vi "Convert_ERDs.vi"(0 "New Header?":bool, 2 "ERD Name":string[](array[string]), 5 "All_Bundled_Data_Brass":T1, 7 "Array":T8[](array[typedef]) {"ERD Number" format="%.0x"}, 11 "Error In":errorcluster) -> (6 "All_ERD_Data_Bundled_Brass":T1, 15 "Error Out":errorcluster)   [LabVIEW 2021]
doc: "This VI parses the data from ERDs in correct format, units, etc. It handles all hex to dec conversions, hex to enum, and hex to boolean conversions.\n\nIf Raw Data from ERD is blank string, then it will output values from shift register."
uses:
  Common/LabVIEW GEA2 Toolkit/GEA3/type defs/ERD Read Data Out.ctl
  Controls/All_Bundled_Data_RT.ctl
  Dryer Tool (Commercial 2)/JL Dryer Tool Support/type defs/Version.ctl
  Dryer Tool (Commercial 2)/JL Dryer Tool Support/type defs/ERD_Always_Show_JL.ctl
  Dryer Tool (Commercial 2)/JL Dryer Tool Support/type defs/CSV_File_String_Arrays.ctl
  Dryer Tool (Commercial 2)/JL Dryer Tool Support/type defs/Fault Table Array.ctl
  Dryer Tool (Commercial 2)/JL Dryer Tool Support/type defs/Fault_Table_Info.ctl
  Dryer Tool (Commercial 2)/JL Dryer Tool Support/type defs/BootloaderVersion.ctl
panel:
  out "Numeric":i32
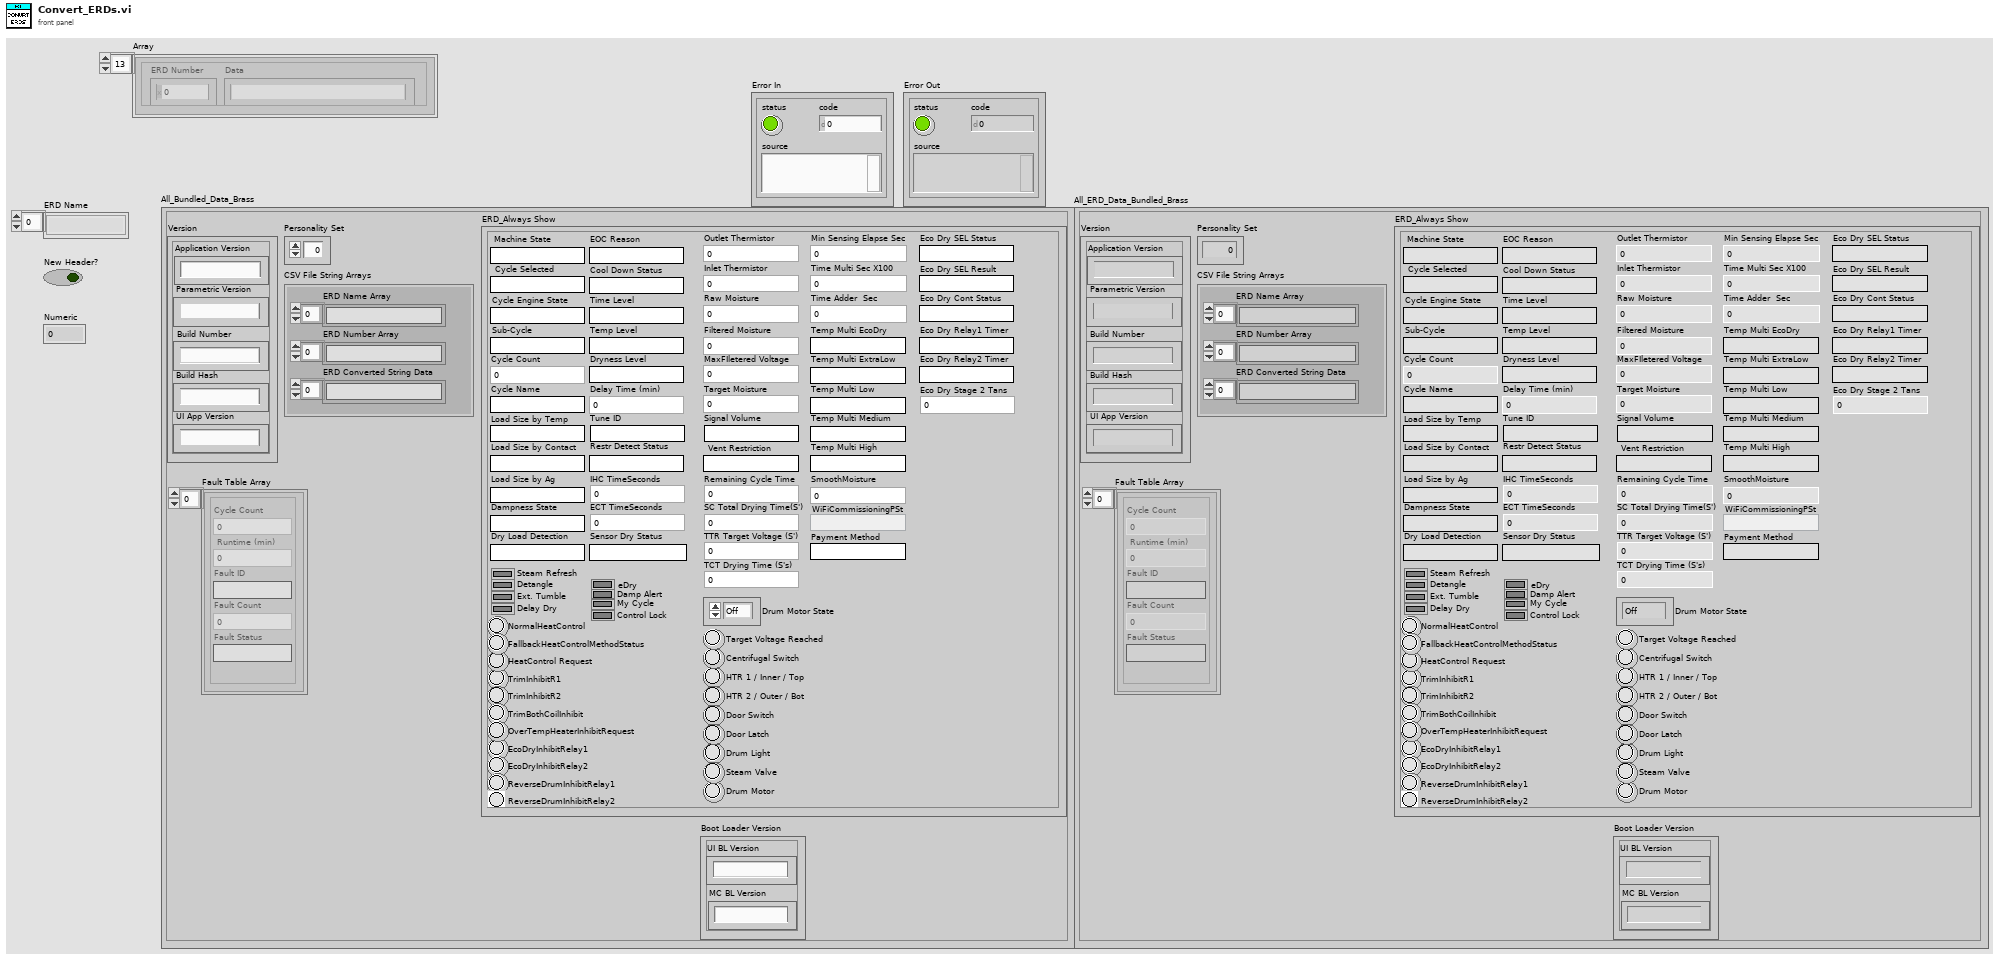
[diagram p1: front panel]
types:
  T1 = typedef "All_Bundled_Data_RT.ctl" = cluster{"Version":T2, "ERD_Always Show":T3, "Personality Set":u8, "CSV File String Arrays":T4, "Fault Table Array ":T5, "Boot Loader Version":T7}
  T2 = typedef "Version.ctl" = cluster{"Build Number":string, "Build Hash ":string, "Application Version":string, "Parametric Version":string, "UI App Version":string}
  T3 = typedef "ERD_Always_Show_JL.ctl" = cluster{"Inlet Thermistor":u16, "Machine State":string, "Filtered Moisture":u16, "Cycle Selected":string, "HTR 1 / Inner / Top":bool, "HTR 2 / Outer / Bot":bool, "Door Switch":bool, "Drum Light":bool, "Cycle Engine State":string, "Centrifugal Switch":bool, "Drum Motor":bool, "Cycle Count":u32, "Ext. Tumble":bool, "eDry":bool, "Temp Level":string, "Dryness Level":string, "Time Level":string, "Delay Time (min)":u16, "Steam Refresh":bool, "Damp Alert":bool, "Sub-Cycle":string, "Outlet Thermistor":u16, "Target Moisture":u16, "Remaining Cycle Time":u32, "Raw Moisture":u16, "Cycle Name":string, "My Cycle":bool, "Delay Dry":bool, "Detangle":bool, "Control Lock":bool, "Steam Valve":bool, "Door Latch":bool, "Signal Volume":string, "Tune ID":string, "Restr Detect Status":string, "Vent Restriction":string, "Load Size by Contact":string, "Load Size by Temp":string, "EOC Reason":string, "Sensor Dry Status":string, "Dampness State":string, "Target Voltage Reached":bool, "TrimInhibitR1":bool, "TrimInhibitR2":bool, "TrimBothCoilInhibit":bool, "NormalHeatControl":bool, "HeatControl Request":bool, "Cool Down Status":string, "EcoDryInhibitRelay1":bool, "EcoDryInhibitRelay2":bool, "ReverseDrumInhibitRelay1":bool, "ReverseDrumInhibitRelay2":bool, "OverTempHeaterInhibitRequest":bool, "FallbackHeatControlMethodStatus":bool, "IHC TimeSeconds":u32, "ECT TimeSeconds ":u32, "SC Total Drying Time(S')":u32, "TTR Target Voltage (S')":u32, "TCT Drying Time (S's)":u32, "Drum Motor State":enum16{"Off", "Cw", "Ccw", "Max"}, "Load Size by Ag":string, "MaxFIletered Voltage":u16, "Dry Load Detection":string, "Min Sensing Elapse Sec":u32, "Time Multi Sec X100":u32, "Time Adder  Sec":u32, "Temp Multi EcoDry":string, "Temp Multi ExtraLow":string, "Temp Multi Low ":string, "Temp Multi Medium":string, "Temp Multi High":string, "SmoothMoisture":u16, "Eco Dry SEL Status":string, "Eco Dry SEL Result":string, "Eco Dry Cont Status":string, "Eco Dry Relay1 Timer":string, "Eco Dry Relay2 Timer ":string, "Eco Dry Stage 2 Tans ":u32, "WiFiCommissioningPSt":string, "Payment Method":string}
  T4 = typedef "CSV_File_String_Arrays.ctl" = cluster{"ERD Number Array":string[], "ERD Name Array":string[], "ERD Converted String Data":string[]}
  T5 = typedef "Fault Table Array.ctl" = T6[]
  T6 = typedef "Fault_Table_Info.ctl" = cluster{"Cycle Count":u32, " Runtime (min) ":u32, "Fault Status":string, "Fault ID":string, "Fault Count":u16}
  T7 = typedef "BootloaderVersion.ctl" = cluster{"UI BL Version":string, "MC BL Version":string}
  T8 = typedef "ERD Read Data Out.ctl" = cluster{"ERD Number":u16, "Data":string}
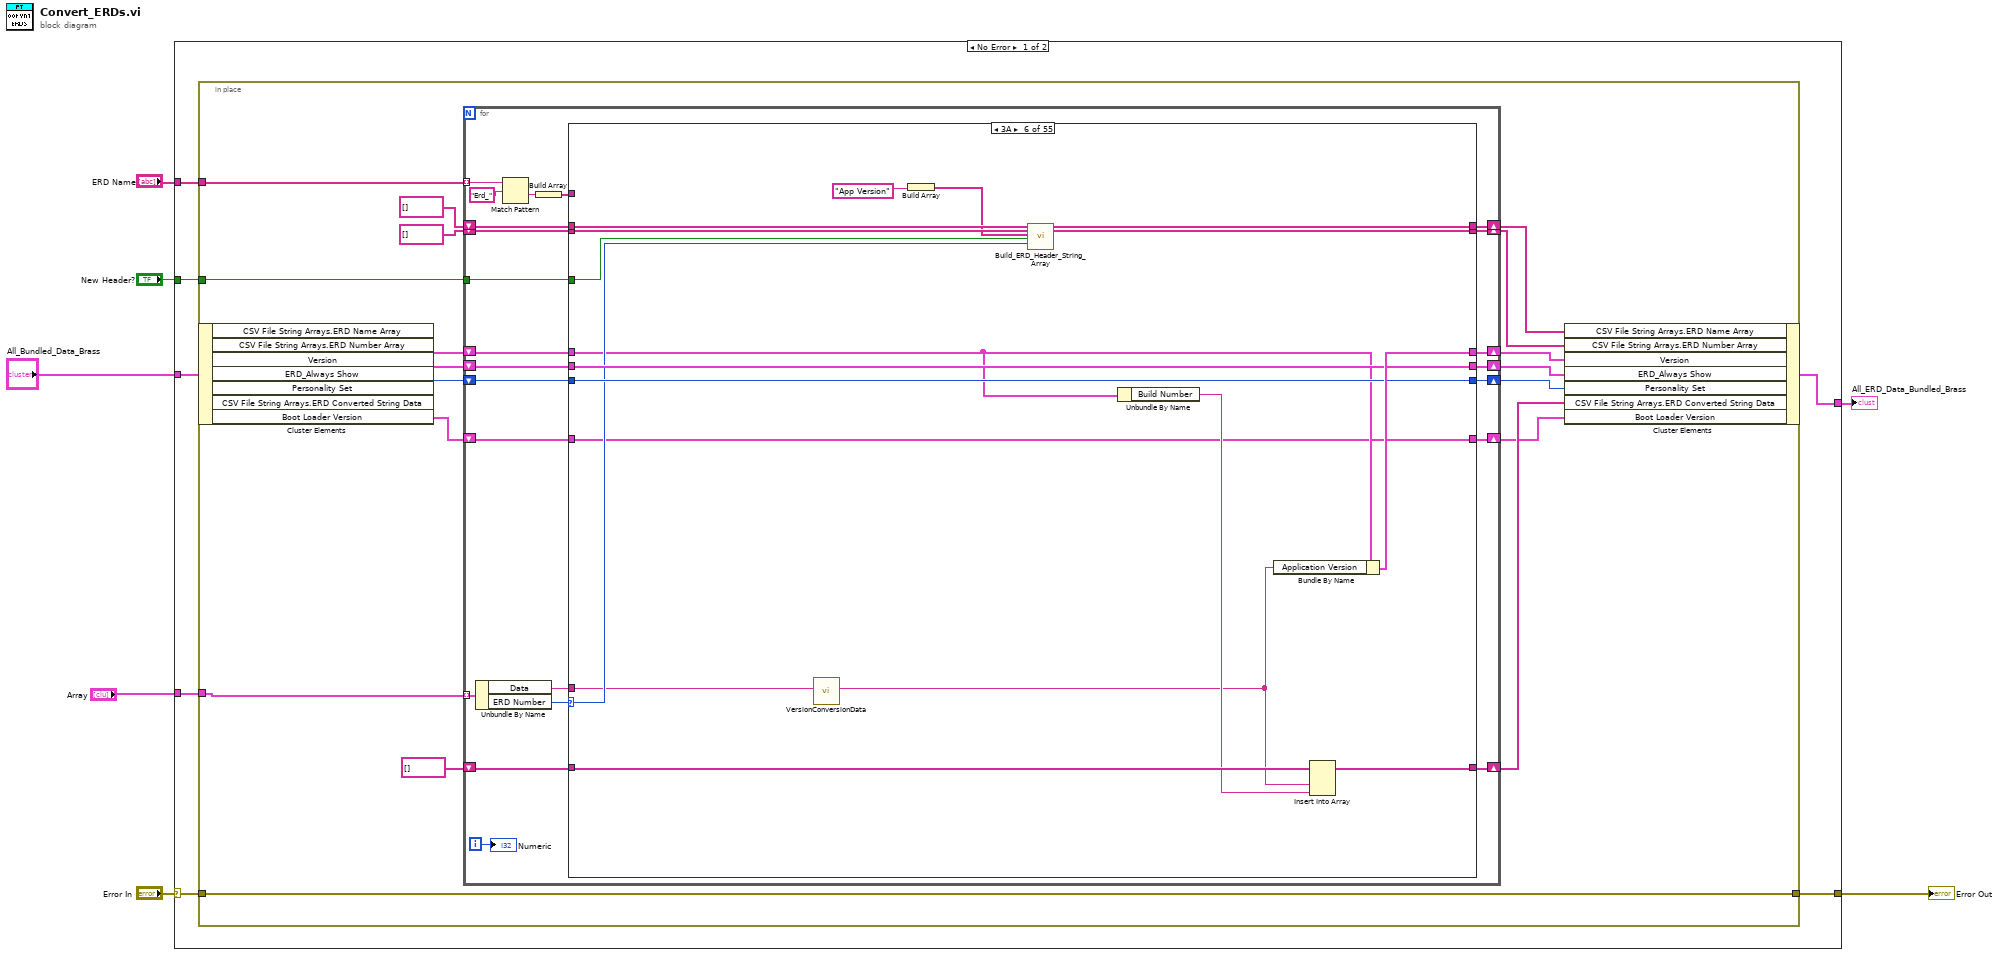
[diagram p0: block diagram]
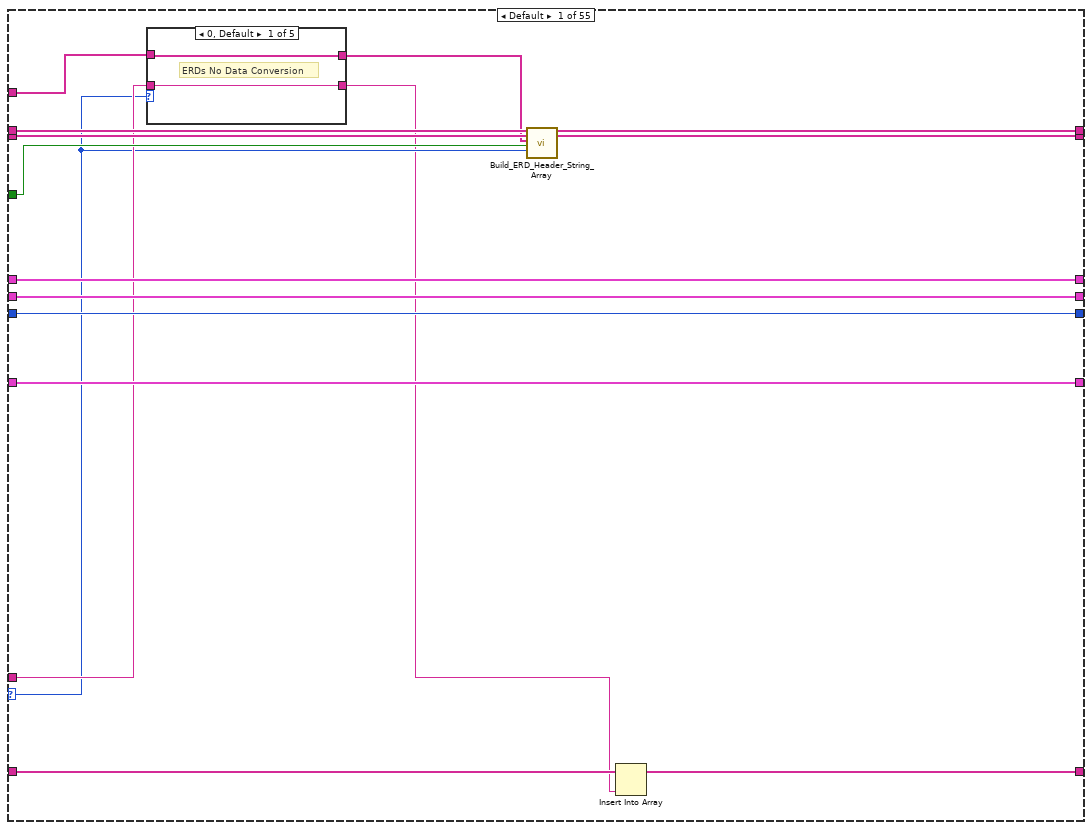
[diagram p2: hidden frame]
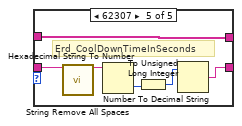
[diagram p6: hidden frame]
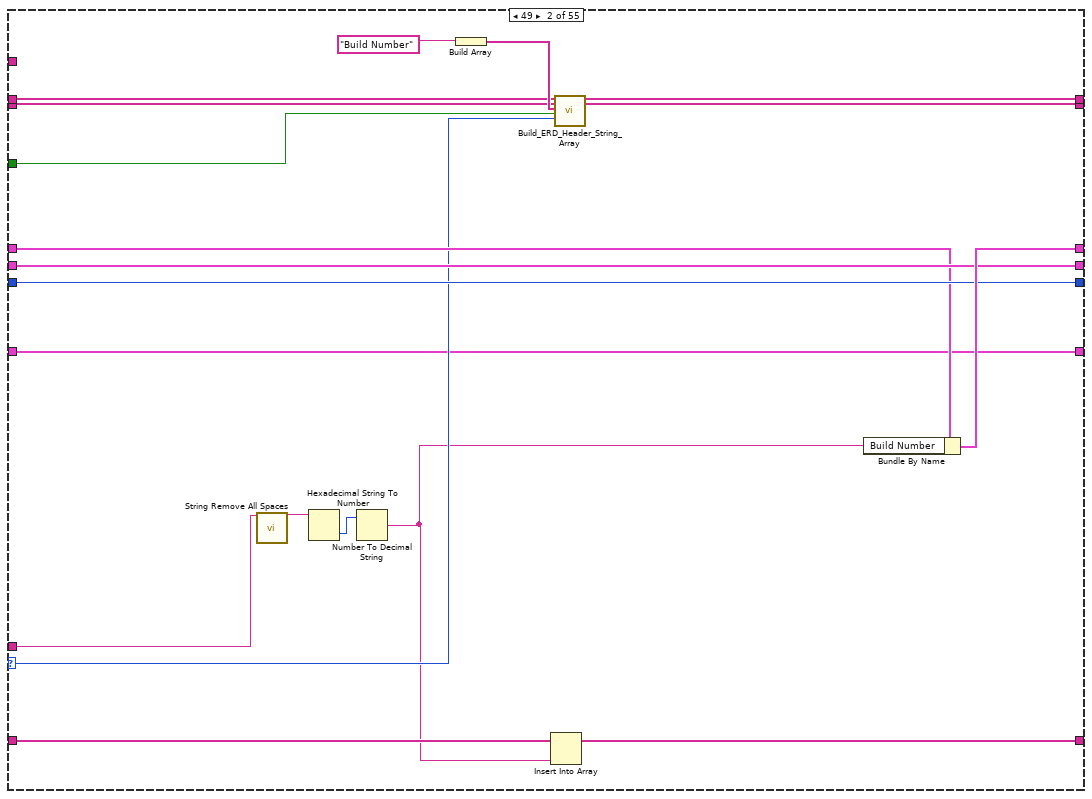
[diagram p7: hidden frame]
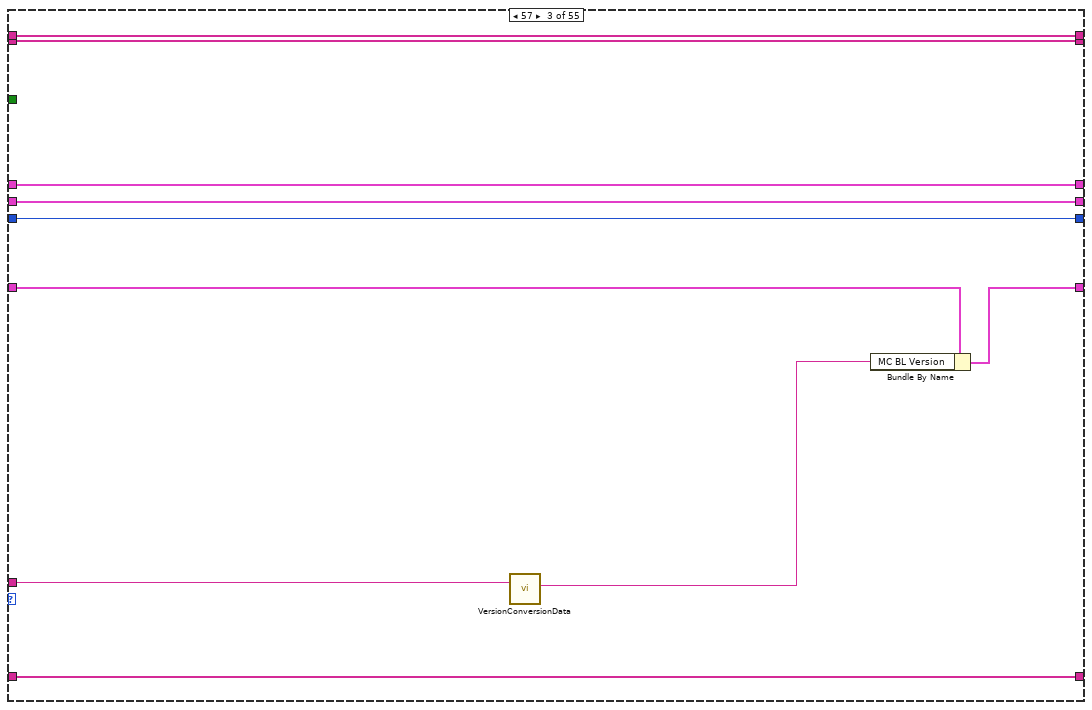
[diagram p8: hidden frame]
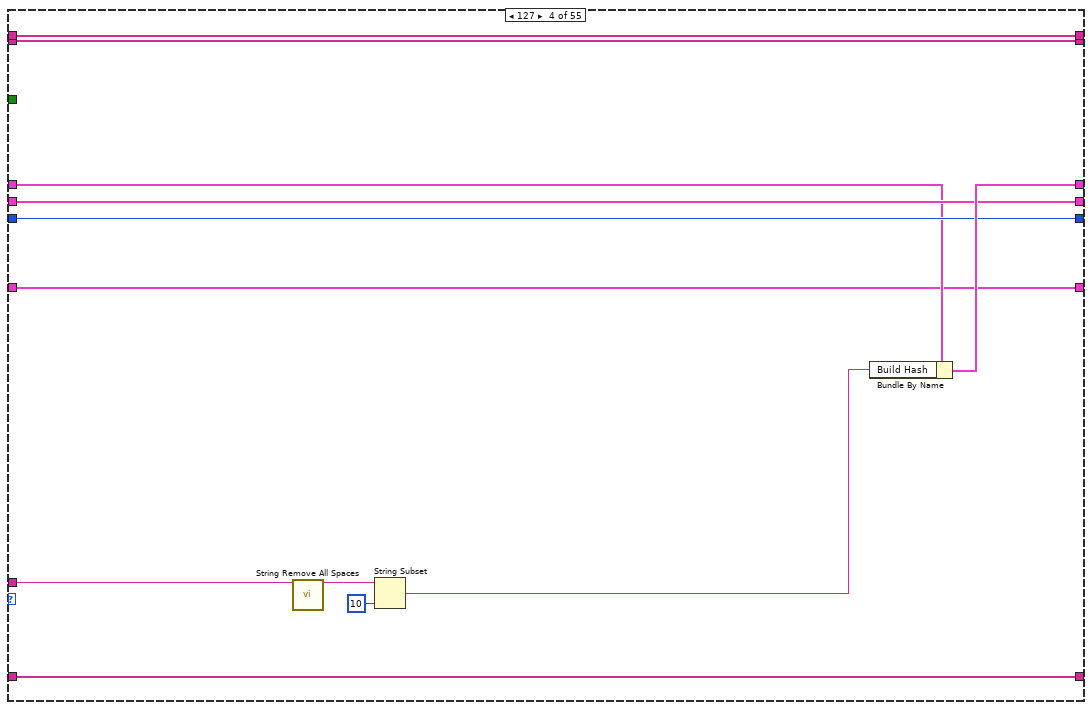
[diagram p9: hidden frame]
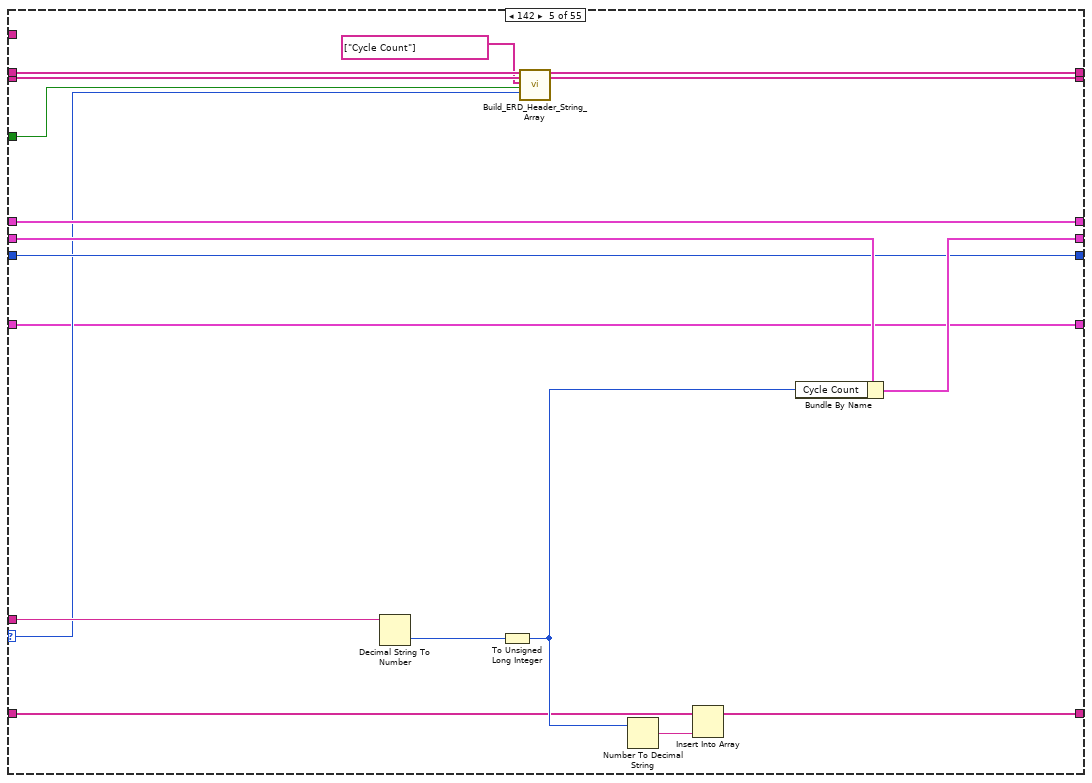
[diagram p10: hidden frame]
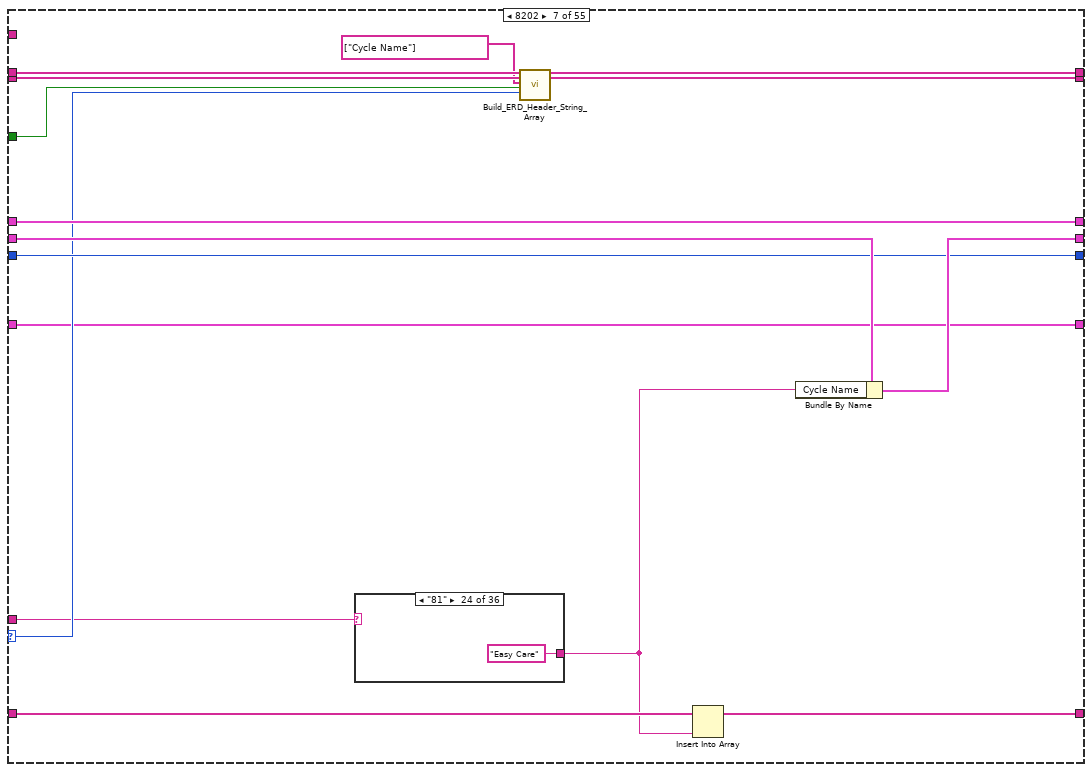
[diagram p11: hidden frame]
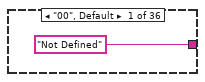
[diagram p12: hidden frame]
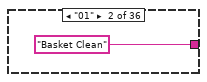
[diagram p13: hidden frame]
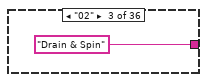
[diagram p14: hidden frame]
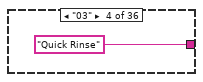
[diagram p15: hidden frame]
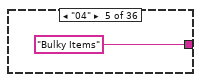
[diagram p16: hidden frame]
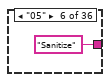
[diagram p17: hidden frame]
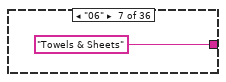
[diagram p18: hidden frame]
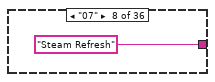
[diagram p19: hidden frame]
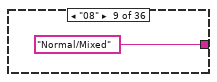
[diagram p20: hidden frame]
diagram:
  n1 = case shown="No Error" "Error In" {
    selector: "Error In" -> [w11 w1202]
    tunnel: "Array" -> [w14 _]
    tunnel: [w12 w1201] -> w5
    tunnel: "All_Bundled_Data_Brass" -> [w13 w1200]
    tunnel: [w10 w1200] -> w1
    tunnel: "New Header?" -> [w9 _]
    tunnel: "ERD Name" -> [w8 _]
    frame No Error {
      n2 = in-place {
        in-place-border: w14 -> [w16]
        in-place-border: [w15] -> w12
        in-place-border: w11 -> [w15]
        in-place-border: w9 -> [w25]
        in-place-border: w8 -> [w17]
        n3 = in-place-cluster #1(w13) -> ("Version"=w31:T2, "ERD_Always Show"=w32:T3, "Personality Set"=w28:u8, "Boot Loader Version"=w19:T7)  [unwired: 3 out]
        n4 = for {
          shift-right: [w54] -> w29
          shift-left: w32 -> [w53]
          shift-right: [w51] -> w30
          shift-left: w31 -> [w52]
          shift-right: [w48] -> w27
          shift-left: w28 -> [w49]
          shift-right: [w46] -> w20
          shift-left: string[] [] ("ERD String Data") -> [w47]
          tunnel: w25 -> [w45]
          shift-right: [w41] -> w21
          shift-left: string[] [] ("ERD String Data") -> [w44]
          shift-right: [w42] -> w22
          shift-left: string[] [] ("ERD String Data") -> [w43]
          shift-right: [w38] -> w18
          shift-left: w19 -> [w39]
          tunnel: w17 -> [w37] mode=indexing
          tunnel: w16 -> [w33] mode=indexing
          i -> [w40]
          n5 = Unbundle By Name(w33) -> ("Data"=w55:string, "ERD Number"=w50:u16)
          n6 = Match Pattern(string=w37, regular expression="Erd_") -> (after substring=w34:string)  [unwired: 1 in, 3 out]
          n7 = Build Array(w34) -> (w35:string[])
          n8 = case shown="3A" w50 {
            selector: w50 -> [w57 w95 _ _ w133 w154 w168 w223 w244 w276 w304 w322 w341 w360 w379 w398 w419 w442 w460 w471 w494 w526 w540 w556 w581 w600 w627 w650 w669 w690 w710 w729 w748 w766 w785 w808 w824 w849 w870 w889 w908 w927 w949 w975 w990 w1014 w1033 w1052 w1074 w1094 w1110 w1133 w1156 w1168 w1192]
            tunnel: w55 -> [w58 w89 w106 w120 w144 w146 w165 w217 w237 w275 w303 w320 w339 w358 w377 w396 w414 w437 w452 w473 w499 w522 w538 w569 w580 w611 w637 w664 w683 w700 w724 w743 w762 w779 w798 w819 w835 w859 w881 w900 w919 w938 w960 w970 w1000 w1013 w1032 w1051 w1085 w1088 w1121 w1131 w1153 w1166 w1184]
            tunnel: [w71 w103 w114 w125 w142 w161 w177 w231 w241 w288 w316 w336 w355 w374 w393 w412 w415 w433 w451 w479 w496 w520 w554 w568 w592 w612 w636 w662 w681 w699 w722 w741 w760 w780 w799 w817 w836 w860 w882 w901 w920 w939 w961 w984 w999 w1026 w1045 w1064 w1083 w1103 w1119 w1127 w1154 w1178 w1185] -> w54
            tunnel: w53 -> [w71 w103 w114 w125 w143 w161 w178 w231 w242 w289 w317 w333 w352 w371 w390 w409 w416 w434 w455 w478 w497 w521 w551 w570 w593 w613 w638 w663 w682 w701 w723 w742 w761 w781 w800 w818 w837 w861 w883 w902 w921 w940 w962 w985 w1001 w1027 w1046 w1065 w1084 w1104 w1120 w1128 w1155 w1178 w1186]
            tunnel: w52 -> [w70 w101 w107 w121 w141 w153 w176 w230 w243 w287 w315 w335 w354 w373 w392 w411 w428 w435 w466 w489 w512 w535 w553 w567 w591 w610 w635 w661 w680 w698 w721 w740 w759 w778 w797 w816 w834 w858 w880 w899 w918 w937 w959 w983 w998 w1025 w1044 w1063 w1082 w1102 w1118 w1141 w1164 w1180 w1196]
            tunnel: [w70 w104 w107 w126 w141 w162 w176 w230 w243 w287 w315 w335 w354 w373 w392 w411 w428 w435 w466 w489 w512 w535 w553 w567 w591 w610 w635 w661 w680 w698 w721 w740 w759 w778 w797 w816 w834 w858 w880 w899 w918 w937 w959 w983 w998 w1025 w1044 w1063 w1082 w1102 w1118 w1141 w1164 w1179 w1196] -> w51
            tunnel: w49 -> [w69 w102 w113 w124 w140 w160 w175 _ w251 w286 w314 w332 w351 w370 w389 w408 w427 w448 w465 w488 w511 w534 w550 w566 w590 w609 w634 w660 w679 w697 w720 w739 w758 w777 w796 w815 w833 w857 w879 w898 w917 w936 w958 w982 w997 w1024 w1043 w1062 w1081 w1101 w1117 w1140 w1163 w1177 w1195]
            tunnel: [w69 w102 w113 w124 w140 w160 w175 w219 w251 w286 w314 w332 w351 w370 w389 w408 w427 w448 w465 w488 w511 w534 w550 w566 w590 w609 w634 w660 w679 w697 w720 w739 w758 w777 w796 w815 w833 w857 w879 w898 w917 w936 w958 w982 w997 w1024 w1043 w1062 w1081 w1101 w1117 w1140 w1163 w1177 w1195] -> w48
            tunnel: w47 -> [w67 w99 w110 w116 w138 w149 w173 w227 w248 w281 w308 w326 w345 w364 w383 w402 w423 w444 w458 w482 w503 w530 w544 w560 w586 w606 w631 w654 w673 w694 w714 w733 w752 w771 w790 w812 w830 w855 w876 w895 w914 w933 w955 w979 w994 w1018 w1037 w1056 w1078 w1098 w1114 w1137 w1160 w1172 w1188]
            tunnel: [w63 w98 w110 w116 w136 w156 w171 w225 w246 w279 w306 w324 w343 w362 w381 w400 w421 w440 w461 w485 w502 w528 w542 w558 w584 w604 w629 w652 w671 w692 w712 w731 w750 w769 w788 w810 w828 w853 w874 w893 w912 w931 w953 w977 w992 w1016 w1035 w1054 w1076 w1096 w1112 w1135 w1158 w1170 w1190] -> w46
            tunnel: w45 -> [w65 w93 _ _ w134 w155 w169 w224 w245 w278 w305 w323 w342 w361 w380 w399 w420 w443 w459 w481 w500 w527 w541 w557 w583 w601 w628 w651 w670 w691 w711 w730 w749 w768 w787 w809 w825 w850 w871 w890 w909 w928 w950 w976 w991 w1015 w1034 w1053 w1075 w1095 w1111 w1134 w1157 w1169 w1193]
            tunnel: w44 -> [w66 w97 w111 w122 w139 w150 w174 w228 w249 w282 w309 w327 w346 w365 w384 w403 w424 w445 w457 w483 w504 w531 w545 w561 w587 w607 w632 w655 w674 w695 w715 w734 w753 w772 w791 w813 w831 w856 w877 w896 w915 w934 w956 w980 w995 w1019 w1038 w1057 w1079 w1099 w1115 w1138 w1161 w1173 w1189]
            tunnel: w43 -> [w61 w91 w112 w123 w129 w159 w167 w221 w234 w284 w312 w330 w349 w368 w387 w406 w418 w439 w453 w476 w498 w524 w548 w565 w589 w603 w626 w658 w677 w689 w718 w737 w756 w775 w794 w807 w827 w852 w873 w892 w911 w930 w952 w974 w989 w1022 w1041 w1060 w1072 w1092 w1109 w1130 w1152 w1176 w1183]
            tunnel: [w62 w90 w112 w123 w128 w158 w166 w220 w233 w283 w311 w329 w348 w367 w386 w405 w417 w438 w454 w477 w495 w525 w547 w564 w588 w602 w625 w657 w676 w688 w717 w736 w755 w774 w793 w806 w826 w851 w872 w891 w910 w929 w951 w973 w988 w1021 w1040 w1059 w1071 w1091 w1108 w1125 w1151 w1175 w1182] -> w42
            tunnel: [w64 w96 w111 w122 w137 w157 w172 w226 w247 w280 w307 w325 w344 w363 w382 w401 w422 w441 w462 w484 w501 w529 w543 w559 w585 w605 w630 w653 w672 w693 w713 w732 w751 w770 w789 w811 w829 w854 w875 w894 w913 w932 w954 w978 w993 w1017 w1036 w1055 w1077 w1097 w1113 w1136 w1159 w1171 w1191] -> w41
            tunnel: w39 -> [w68 w92 w109 w115 w127 w151 w163 w218 w232 w273 w294 w318 w337 w356 w375 w394 w426 w447 w464 w487 w510 w533 w536 w555 w578 w598 w623 w648 w667 w686 w708 w727 w746 w765 w784 w803 w822 w847 w868 w887 w906 w925 w947 w967 w986 w1011 w1030 w1049 w1068 w1086 w1105 w1139 w1149 w1167 w1194]
            tunnel: [w68 w92 w108 w115 w127 w151 w163 w218 w232 w273 w294 w318 w337 w356 w375 w394 w426 w447 w464 w487 w510 w533 w536 w555 w578 w598 w623 w648 w667 w686 w708 w727 w746 w765 w784 w803 w822 w847 w868 w887 w906 w925 w947 w967 w986 w1011 w1030 w1049 w1068 w1086 w1105 w1139 w1149 w1167 w1194] -> w38
            tunnel: w35 -> [w59 _ _ _ _ _ _ w215 _ _ _ _ _ _ _ _ _ _ _ _ _ _ _ _ _ _ _ _ _ _ _ _ _ _ _ _ _ w846 _ _ _ _ _ _ _ _ _ _ _ _ _ w1124 _ _ w1187]
            frame Default {
              n9 = case shown="0, Default" w57 {
                tunnel: [w72 w75 w77 w79 w85] -> w60
                tunnel: w59 -> [w72 w75 w77 w79 w85]
                tunnel: w58 -> [w73 w74 w76 w78 w82]
                tunnel: [w73 w74 w76 w78 w80] -> w56
                frame 0, Default {
                  # "ERDs No Data Conversion"
                }
                frame 65423 {
                  # "Consumer Error Mode"
                }
                frame 55 {
                  # "ServiceModeState"
                }
                frame 61811 {
                  # "WiFiCommissioningOption"
                }
                frame 62307 {
                  # "Erd_CoolDownTimeInSeconds"
                  n10 = call "String Remove All Spaces.vi"("Input String"=w82) -> ("Spaces Removed"=w83:string)  [unwired: 13 in, 1 out]
                  n11 = Hexadecimal String To Number(string=w83) -> (number=w84:u32)  [unwired: 2 in, 1 out]
                  n12 = To Unsigned Long Integer(number=w84) -> (unsigned 32bit integer=w81:u32)
                  n13 = Number To Decimal String(number=w81) -> (decimal integer string=w80:string)  [unwired: 1 in]
                }
              }
              n14 = call "Build_ERD_Header_String_Array.vi"("ERD Name Array In"=w66, "ERD Number Array In"=w67, "ERD Name List"=w60, "New Header?"=w65, "ERD Number"=w57) -> ("ERD Name Array Out"=w64:string[], "ERD Number Array Out"=w63:string[])  [unwired: 13 in]
              n15 = Insert Into Array(array=w61, new element=w56) -> (w62:string[])  [unwired: 1 in]
            }
            frame 49 {
              n16 = call "String Remove All Spaces.vi"("Input String"=w89) -> ("Spaces Removed"=w88:string)  [unwired: 13 in, 1 out]
              n17 = Hexadecimal String To Number(string=w88) -> (number=w86:u32)  [unwired: 2 in, 1 out]
              n18 = Number To Decimal String(number=w86) -> (decimal integer string=w87:string)  [unwired: 1 in]
              n19 = Build Array("Build Number") -> (w100:string[])
              n20 = Insert Into Array(array=w91, new element=w87) -> (w90:string[])  [unwired: 1 in]
              n21 = call "Build_ERD_Header_String_Array.vi"("ERD Name Array In"=w97, "ERD Number Array In"=w99, "ERD Name List"=w100, "New Header?"=w93, "ERD Number"=w95) -> ("ERD Name Array Out"=w96:string[], "ERD Number Array Out"=w98:string[])  [unwired: 13 in]
              n22 = Bundle By Name(cluster=w101, "Build Number"=w87) -> (w104:T2)
            }
            frame 57 {
              n23 = call "VersionConversionData.vi"("Version In"=w106) -> ("Version Out"=w105:string)  [unwired: 9 in, 1 out]
              n24 = Bundle By Name(cluster=w109, "MC BL Version"=w105) -> (w108:T7)
            }
            frame 127 {
              n25 = call "String Remove All Spaces.vi"("Input String"=w120) -> ("Spaces Removed"=w119:string)  [unwired: 13 in, 1 out]
              n26 = String Subset(string=w119, length (rest)=10 ("length (rest)")) -> (substring=w117:string)  [unwired: 1 in]
              n27 = Bundle By Name(cluster=w121, "Build Hash"=w117) -> (w126:T2)
            }
            frame 142 {
              n28 = Decimal String To Number(string=w144) -> (number=w131:i32)  [unwired: 2 in, 1 out]
              n29 = To Unsigned Long Integer(number=w131) -> (unsigned 32bit integer=w130:u32)
              n30 = call "Build_ERD_Header_String_Array.vi"("ERD Name Array In"=w139, "ERD Number Array In"=w138, "ERD Name List"=string[] ["Cycle Count"], "New Header?"=w134, "ERD Number"=w133) -> ("ERD Name Array Out"=w137:string[], "ERD Number Array Out"=w136:string[])  [unwired: 13 in]
              n31 = Number To Decimal String(number=w130) -> (decimal integer string=w132:string)  [unwired: 1 in]
              n32 = Insert Into Array(array=w129, new element=w132) -> (w128:string[])  [unwired: 1 in]
              n33 = Bundle By Name(cluster=w143, "Cycle Count"=w130) -> (w142:T3)
            }
            frame 58 {
              n34 = call "VersionConversionData.vi"("Version In"=w146) -> ("Version Out"=w145:string)  [unwired: 9 in, 1 out]
              n35 = Build Array("App Version" ("String")) -> (w147:string[])
              n36 = call "Build_ERD_Header_String_Array.vi"("ERD Name Array In"=w150, "ERD Number Array In"=w149, "ERD Name List"=w147, "New Header?"=w155, "ERD Number"=w154) -> ("ERD Name Array Out"=w157:string[], "ERD Number Array Out"=w156:string[])  [unwired: 13 in]
              n37 = Unbundle By Name(w153) -> ("Build Number"=w152:string)
              n38 = Bundle By Name(cluster=w153, "Application Version"=w145) -> (w162:T2)
              n39 = Insert Into Array(array=w159, new element #1=w145, new element #2=w152) -> (w158:string[])  [unwired: 1 in]
            }
            frame 8202 {
              n40 = case shown="\"81\"" w165 {
                tunnel: ["Not Defined" "Basket Clean" "Drain & Spin" "Quick Rinse" "Bulky Items" "Sanitize" "Towels & Sheets" "Steam Refresh" "Normal/Mixed" "Whites" "Dark Colors" "Jeans" "Hand Wash" "Delicates" "Speed Wash" "Heavy Duty" "Allergen" "Power Clean" "Rinse & Spin" "Single Item" "Colors" "Cold Wash" "Cottons" "Easy Care" "Active Wear" "Timed Dry" "Dewrinkle" "Air Fluff" "Steam Refresh" "Steam Dewrinkle" "Speed Dry" "Mixed" "Quick Dry" "Casuals" "Warm Up" "Energy Saver"] -> w164
                frame "00", Default {
                }
                frame "01" {
                }
                frame "02" {
                }
                frame "03" {
                }
                frame "04" {
                }
                frame "05" {
                }
                frame "06" {
                }
                frame "07" {
                }
                frame "08" {
                }
                frame "09" {
                }
                frame "0A" {
                }
                frame "0B" {
                }
                frame "0C" {
                }
                frame "0D" {
                }
                frame "0E" {
                }
                frame "0F" {
                }
                frame "10" {
                }
                frame "11" {
                }
                frame "12" {
                }
                frame "13" {
                }
                frame "14" {
                }
                frame "15" {
                }
                frame "80" {
                }
                frame "81" {
                }
                frame "82" {
                }
                frame "83" {
                }
                frame "84" {
                }
                frame "85" {
                }
                frame "86" {
                }
                frame "87" {
                }
                frame "88" {
                }
                frame "89" {
                }
                frame "8A" {
                }
                frame "8B" {
                }
                frame "8C" {
                }
                frame "8D" {
                }
              }
              n41 = call "Build_ERD_Header_String_Array.vi"("ERD Name Array In"=w174, "ERD Number Array In"=w173, "ERD Name List"=string[] ["Cycle Name"], "New Header?"=w169, "ERD Number"=w168) -> ("ERD Name Array Out"=w172:string[], "ERD Number Array Out"=w171:string[])  [unwired: 13 in]
              n42 = Insert Into Array(array=w167, new element=w164) -> (w166:string[])  [unwired: 1 in]
              n43 = Bundle By Name(cluster=w178, "Cycle Name"=w164) -> (w177:T3)
            }
            frame 65281 {
              n44 = call "String Remove All Spaces.vi"("Input String"=w217) -> ("Spaces Removed"=w216:string)  [unwired: 13 in, 1 out]
              n45 = Decimal String To Number(string=w216) -> (number=w229:i32)  [unwired: 2 in, 1 out]
              n46 = To Unsigned Byte Integer(number=w229) -> (unsigned 8bit integer=w219:u8)
              n47 = call "Build_ERD_Header_String_Array.vi"("ERD Name Array In"=w228, "ERD Number Array In"=w227, "ERD Name List"=w215, "New Header?"=w224, "ERD Number"=w223) -> ("ERD Name Array Out"=w226:string[], "ERD Number Array Out"=w225:string[])  [unwired: 13 in]
              n48 = Number To Decimal String(number=w219) -> (decimal integer string=w222:string)  [unwired: 1 in]
              n49 = Insert Into Array(array=w221, new element=w222) -> (w220:string[])  [unwired: 1 in]
            }
            frame 61443 {
              n50 = String Subset(string=w237, offset (0)=3, length (rest)=2 ("length (rest)")) -> (substring=w238:string)
              n51 = Hexadecimal String To Number(string=w238) -> (number=w236:u32)  [unwired: 2 in, 1 out]
              n52 = case shown="4" w236 {
                tunnel: ["Warning" ("Motor Profile") "Power Up" ("Motor Profile") "Power Down" ("Motor Profile") "Increase Sound" ("Motor Profile") "Decrease Sound" ("Motor Profile") "OK" ("Motor Profile") "OK Volume Key" ("Motor Profile") "Unavailable" ("Motor Profile") "Knob Turn" ("Motor Profile") "Notification 1" ("Motor Profile") "Notification 2" ("Motor Profile") "Notification 3" ("Motor Profile") "Notification Intro" ("Motor Profile") "Notification End" ("Motor Profile") "Feature ON" ("Motor Profile") "Feature OFF" ("Motor Profile") "Hold ON" ("Motor Profile") "Hold ON Volume" ("Motor Profile") "Hold OFF" ("Motor Profile") "Max" ("Motor Profile") "none" ("Motor Profile")] -> w235
                frame 0, Default {
                }
                frame 1 {
                }
                frame 2 {
                }
                frame 3 {
                }
                frame 4 {
                }
                frame 5 {
                }
                frame 6 {
                }
                frame 7 {
                }
                frame 8 {
                }
                frame 9 {
                }
                frame 10 {
                }
                frame 11 {
                }
                frame 12 {
                }
                frame 13 {
                }
                frame 14 {
                }
                frame 15 {
                }
                frame 16 {
                }
                frame 17 {
                }
                frame 18 {
                }
                frame 19 {
                }
                frame 20 {
                }
              }
              n53 = call "Build_ERD_Header_String_Array.vi"("ERD Name Array In"=w249, "ERD Number Array In"=w248, "ERD Name List"=string[] ["Tune ID"], "New Header?"=w245, "ERD Number"=w244) -> ("ERD Name Array Out"=w247:string[], "ERD Number Array Out"=w246:string[])  [unwired: 13 in]
              n54 = Insert Into Array(array=w234, new element=w235) -> (w233:string[])  [unwired: 1 in]
              n55 = Bundle By Name(cluster=w242, "Tune ID"=w235) -> (w241:T3)
            }
            frame 8323 {
              n56 = case shown="\"02\"" w275 {
                tunnel: [FALSE TRUE] -> w274
                frame "01", Default {
                }
                frame "02" {
                }
              }
              n57 = case shown="True" w274 {
                tunnel: ["OFF" "ON"] -> w285
                frame False {
                }
                frame True {
                }
              }
              n58 = call "Build_ERD_Header_String_Array.vi"("ERD Name Array In"=w282, "ERD Number Array In"=w281, "ERD Name List"=string[] ["Control Lock"], "New Header?"=w278, "ERD Number"=w276) -> ("ERD Name Array Out"=w280:string[], "ERD Number Array Out"=w279:string[])  [unwired: 13 in]
              n59 = Insert Into Array(array=w284, new element=w285) -> (w283:string[])  [unwired: 1 in]
              n60 = Bundle By Name(cluster=w289, "Control Lock"=w274) -> (w288:T3)
            }
            frame 61478 {
              n61 = String Subset(string=w303, length (rest)=11 ("length (rest)")) -> (substring=w301:string)  [unwired: 1 in]
              n62 = call "String Remove All Spaces.vi"("Input String"=w301) -> ("Spaces Removed"=w300:string)  [unwired: 13 in, 1 out]
              n63 = Hexadecimal String To Number(string=w300) -> (number=w299:u32)  [unwired: 2 in, 1 out]
              n64 = To Double Precision Float(number=w299) -> (double precision float=w296:dbl)
              n65 = Divide(x=w296, y=60.0) -> (x/y=w298:dbl)
              n66 = call "Build_ERD_Header_String_Array.vi"("ERD Name Array In"=w309, "ERD Number Array In"=w308, "ERD Name List"=string[] ["Delay Time"], "New Header?"=w305, "ERD Number"=w304) -> ("ERD Name Array Out"=w307:string[], "ERD Number Array Out"=w306:string[])  [unwired: 13 in]
              n67 = To Unsigned Word Integer(number=w298) -> (unsigned 16bit integer=w297:u16)
              n68 = Number To Decimal String(number=w297) -> (decimal integer string=w313:string)  [unwired: 1 in]
              n69 = Bundle By Name(cluster=w317, "Delay Time (min)"=w297) -> (w316:T3)
              n70 = Insert Into Array(array=w312, new element=w313) -> (w311:string[])  [unwired: 1 in]
            }
            frame 61479 {
              n71 = call "String Remove All Spaces.vi"("Input String"=w320) -> ("Spaces Removed"=w319:string)  [unwired: 13 in, 1 out]
              n72 = Hexadecimal String To Number(string=w319) -> (number=w334:u32)  [unwired: 2 in, 1 out]
              n73 = To Unsigned Long Integer(number=w334) -> (unsigned 32bit integer=w321:u32)
              n74 = Bundle By Name(cluster=w333, "Remaining Cycle Time"=w321) -> (w336:T3)
              n75 = Number To Decimal String(number=w321) -> (decimal integer string=w331:string)  [unwired: 1 in]
              n76 = call "Build_ERD_Header_String_Array.vi"("ERD Name Array In"=w327, "ERD Number Array In"=w326, "ERD Name List"=string[] ["Remaing Cycle Time"], "New Header?"=w323, "ERD Number"=w322) -> ("ERD Name Array Out"=w325:string[], "ERD Number Array Out"=w324:string[])  [unwired: 13 in]
              n77 = Insert Into Array(array=w330, new element=w331) -> (w329:string[])  [unwired: 1 in]
            }
            frame 61698 {
              n78 = call "String Remove All Spaces.vi"("Input String"=w339) -> ("Spaces Removed"=w338:string)  [unwired: 13 in, 1 out]
              n79 = Hexadecimal String To Number(string=w338) -> (number=w353:u32)  [unwired: 2 in, 1 out]
              n80 = To Unsigned Long Integer(number=w353) -> (unsigned 32bit integer=w340:u32)
              n81 = Bundle By Name(cluster=w352, "IHC TimeSeconds"=w340) -> (w355:T3)
              n82 = Number To Decimal String(number=w340) -> (decimal integer string=w350:string)  [unwired: 1 in]
              n83 = call "Build_ERD_Header_String_Array.vi"("ERD Name Array In"=w346, "ERD Number Array In"=w345, "ERD Name List"=string[] ["Init HeatingTime Sec"], "New Header?"=w342, "ERD Number"=w341) -> ("ERD Name Array Out"=w344:string[], "ERD Number Array Out"=w343:string[])  [unwired: 13 in]
              n84 = Insert Into Array(array=w349, new element=w350) -> (w348:string[])  [unwired: 1 in]
            }
            frame 61606 {
              n85 = call "String Remove All Spaces.vi"("Input String"=w358) -> ("Spaces Removed"=w357:string)  [unwired: 13 in, 1 out]
              n86 = Hexadecimal String To Number(string=w357) -> (number=w372:u32)  [unwired: 2 in, 1 out]
              n87 = To Unsigned Long Integer(number=w372) -> (unsigned 32bit integer=w359:u32)
              n88 = Bundle By Name(cluster=w371, "ECT TimeSeconds"=w359) -> (w374:T3)
              n89 = Number To Decimal String(number=w359) -> (decimal integer string=w369:string)  [unwired: 1 in]
              n90 = call "Build_ERD_Header_String_Array.vi"("ERD Name Array In"=w365, "ERD Number Array In"=w364, "ERD Name List"=string[] ["Elapsed Cycle Time Sec"], "New Header?"=w361, "ERD Number"=w360) -> ("ERD Name Array Out"=w363:string[], "ERD Number Array Out"=w362:string[])  [unwired: 13 in]
              n91 = Insert Into Array(array=w368, new element=w369) -> (w367:string[])  [unwired: 1 in]
            }
            frame 61607 {
              n92 = call "String Remove All Spaces.vi"("Input String"=w377) -> ("Spaces Removed"=w376:string)  [unwired: 13 in, 1 out]
              n93 = Hexadecimal String To Number(string=w376) -> (number=w391:u32)  [unwired: 2 in, 1 out]
              n94 = To Unsigned Long Integer(number=w391) -> (unsigned 32bit integer=w378:u32)
              n95 = Bundle By Name(cluster=w390, "SC Total Drying Time(S')"=w378) -> (w393:T3)
              n96 = Number To Decimal String(number=w378) -> (decimal integer string=w388:string)  [unwired: 1 in]
              n97 = call "Build_ERD_Header_String_Array.vi"("ERD Name Array In"=w384, "ERD Number Array In"=w383, "ERD Name List"=string[] ["Sensing Ccle Total Drying Time sec"], "New Header?"=w380, "ERD Number"=w379) -> ("ERD Name Array Out"=w382:string[], "ERD Number Array Out"=w381:string[])  [unwired: 13 in]
              n98 = Insert Into Array(array=w387, new element=w388) -> (w386:string[])  [unwired: 1 in]
            }
            frame 61628 {
              n99 = call "String Remove All Spaces.vi"("Input String"=w396) -> ("Spaces Removed"=w395:string)  [unwired: 13 in, 1 out]
              n100 = Hexadecimal String To Number(string=w395) -> (number=w410:u32)  [unwired: 2 in, 1 out]
              n101 = To Unsigned Long Integer(number=w410) -> (unsigned 32bit integer=w397:u32)
              n102 = Bundle By Name(cluster=w409, "TTR Target Voltage (S')"=w397) -> (w412:T3)
              n103 = Number To Decimal String(number=w397) -> (decimal integer string=w407:string)  [unwired: 1 in]
              n104 = call "Build_ERD_Header_String_Array.vi"("ERD Name Array In"=w403, "ERD Number Array In"=w402, "ERD Name List"=string[] ["TTRTVoltage Seconds"], "New Header?"=w399, "ERD Number"=w398) -> ("ERD Name Array Out"=w401:string[], "ERD Number Array Out"=w400:string[])  [unwired: 13 in]
              n105 = Insert Into Array(array=w406, new element=w407) -> (w405:string[])  [unwired: 1 in]
            }
            frame 61728 {
              n106 = case shown="\"03\"" w414 {
                tunnel: ["Disabled" "Enabled" "Detect" "Finished"] -> w413
                frame "00", Default {
                }
                frame "01" {
                }
                frame "02" {
                }
                frame "03" {
                }
              }
              n107 = call "Build_ERD_Header_String_Array.vi"("ERD Name Array In"=w424, "ERD Number Array In"=w423, "ERD Name List"=string[] ["Eco Dry Sensor Dry Selector Status"], "New Header?"=w420, "ERD Number"=w419) -> ("ERD Name Array Out"=w422:string[], "ERD Number Array Out"=w421:string[])  [unwired: 13 in]
              n108 = Insert Into Array(array=w418, new element=w413) -> (w417:string[])  [unwired: 1 in]
              n109 = Bundle By Name(cluster=w416, "Eco Dry SEL Status"=w413) -> (w415:T3)
            }
            frame 61729 {
              n110 = case shown="\"00\", Default" w437 {
                tunnel: ["NormalDOD" "EDryDOD"] -> w436
                frame "00", Default {
                }
                frame "01" {
                }
              }
              n111 = call "Build_ERD_Header_String_Array.vi"("ERD Name Array In"=w445, "ERD Number Array In"=w444, "ERD Name List"=string[] ["Eco Dry Sensor Dry Selector Status"], "New Header?"=w443, "ERD Number"=w442) -> ("ERD Name Array Out"=w441:string[], "ERD Number Array Out"=w440:string[])  [unwired: 13 in]
              n112 = Insert Into Array(array=w439, new element=w436) -> (w438:string[])  [unwired: 1 in]
              n113 = Bundle By Name(cluster=w434, "Eco Dry SEL Result"=w436) -> (w433:T3)
            }
            frame 61736 {
              n114 = case shown="\"03\"" w452 {
                tunnel: ["Disabled" "Idle" "EcoDry Stage 1" "EcoDry Stage 2"] -> w456
                frame "00", Default {
                }
                frame "01" {
                }
                frame "02" {
                }
                frame "03" {
                }
              }
              n115 = call "Build_ERD_Header_String_Array.vi"("ERD Name Array In"=w457, "ERD Number Array In"=w458, "ERD Name List"=string[] ["Eco Dry Cont Status"], "New Header?"=w459, "ERD Number"=w460) -> ("ERD Name Array Out"=w462:string[], "ERD Number Array Out"=w461:string[])  [unwired: 13 in]
              n116 = Insert Into Array(array=w453, new element=w456) -> (w454:string[])  [unwired: 1 in]
              n117 = Bundle By Name(cluster=w455, "Eco Dry Cont Status"=w456) -> (w451:T3)
            }
            frame 61737 {
              n118 = String Subset(string=w473, offset (0)=12, length (rest)=2 ("length (rest)")) -> (substring=w472:string)
              n119 = case shown="\"03\"" w472 {
                tunnel: ["Disabled" "Not Inhibiting" "Active Inhibiting" "Max"] -> w480
                frame "00", Default {
                }
                frame "01" {
                }
                frame "02" {
                }
                frame "03" {
                }
              }
              n120 = call "Build_ERD_Header_String_Array.vi"("ERD Name Array In"=w483, "ERD Number Array In"=w482, "ERD Name List"=string[] ["Eco Dry Relay1 Timer"], "New Header?"=w481, "ERD Number"=w471) -> ("ERD Name Array Out"=w484:string[], "ERD Number Array Out"=w485:string[])  [unwired: 13 in]
              n121 = Bundle By Name(cluster=w478, "Eco Dry Relay1 Timer"=w480) -> (w479:T3)
              n122 = Insert Into Array(array=w476, new element=w480) -> (w477:string[])  [unwired: 1 in]
            }
            frame 61738 {
              n123 = String Subset(string=w499, offset (0)=12, length (rest)=2 ("length (rest)")) -> (substring=w505:string)
              n124 = case shown="\"03\"" w505 {
                tunnel: ["Disabled" "Not Inhibiting" "Active Inhibiting" "Max"] -> w508
                frame "00", Default {
                }
                frame "01" {
                }
                frame "02" {
                }
                frame "03" {
                }
              }
              n125 = call "Build_ERD_Header_String_Array.vi"("ERD Name Array In"=w504, "ERD Number Array In"=w503, "ERD Name List"=string[] ["Eco Dry Relay2 Timer"], "New Header?"=w500, "ERD Number"=w494) -> ("ERD Name Array Out"=w501:string[], "ERD Number Array Out"=w502:string[])  [unwired: 13 in]
              n126 = Bundle By Name(cluster=w497, "Eco Dry Relay2 Timer"=w508) -> (w496:T3)
              n127 = Insert Into Array(array=w498, new element=w508) -> (w495:string[])  [unwired: 1 in]
            }
            frame 61739 {
              n128 = call "String Remove All Spaces.vi"("Input String"=w522) -> ("Spaces Removed"=w518:string)  [unwired: 13 in, 1 out]
              n129 = Hexadecimal String To Number(string=w518) -> (number=w523:u32)  [unwired: 2 in, 1 out]
              n130 = To Unsigned Long Integer(number=w523) -> (unsigned 32bit integer=w517:u32)
              n131 = call "Build_ERD_Header_String_Array.vi"("ERD Name Array In"=w531, "ERD Number Array In"=w530, "ERD Name List"=string[] ["Eco Dry  Stage 2 Trans"], "New Header?"=w527, "ERD Number"=w526) -> ("ERD Name Array Out"=w529:string[], "ERD Number Array Out"=w528:string[])  [unwired: 13 in]
              n132 = Number To Decimal String(number=w517) -> (decimal integer string=w519:string)  [unwired: 1 in]
              n133 = Bundle By Name(cluster=w521, "Eco Dry Stage 2 Tans"=w517) -> (w520:T3)
              n134 = Insert Into Array(array=w524, new element=w519) -> (w525:string[])  [unwired: 1 in]
            }
            frame 61563 {
              n135 = call "String Remove All Spaces.vi"("Input String"=w538) -> ("Spaces Removed"=w537:string)  [unwired: 13 in, 1 out]
              n136 = Hexadecimal String To Number(string=w537) -> (number=w552:u32)  [unwired: 2 in, 1 out]
              n137 = To Unsigned Long Integer(number=w552) -> (unsigned 32bit integer=w539:u32)
              n138 = Bundle By Name(cluster=w551, "TCT Drying Time (S's)"=w539) -> (w554:T3)
              n139 = Number To Decimal String(number=w539) -> (decimal integer string=w549:string)  [unwired: 1 in]
              n140 = call "Build_ERD_Header_String_Array.vi"("ERD Name Array In"=w545, "ERD Number Array In"=w544, "ERD Name List"=string[] ["Timed Cycle Total Drying Time Seconds"], "New Header?"=w541, "ERD Number"=w540) -> ("ERD Name Array Out"=w543:string[], "ERD Number Array Out"=w542:string[])  [unwired: 13 in]
              n141 = Insert Into Array(array=w548, new element=w549) -> (w547:string[])  [unwired: 1 in]
            }
            frame 61480 {
              n142 = case shown="\"08\"" w569 {
                selector: w569 -> [w571 _ _ _ _ _ _]
                tunnel: [w571 "NONE" "FILL" "SOAK" "WASH" "RINSE" "SPIN"] -> w563
                frame Default {
                }
                frame "00" {
                }
                frame "01" {
                }
                frame "02" {
                }
                frame "04" {
                }
                frame "08" {
                }
                frame "10" {
                }
              }
              n143 = call "Build_ERD_Header_String_Array.vi"("ERD Name Array In"=w561, "ERD Number Array In"=w560, "ERD Name List"=string[] ["Sub-Cycle"], "New Header?"=w557, "ERD Number"=w556) -> ("ERD Name Array Out"=w559:string[], "ERD Number Array Out"=w558:string[])  [unwired: 13 in]
              n144 = Insert Into Array(array=w565, new element=w563) -> (w564:string[])  [unwired: 1 in]
              n145 = Bundle By Name(cluster=w570, "Sub-Cycle"=w563) -> (w568:T3)
            }
            frame 61483 {
              n146 = case shown="\"02\"" w580 {
                tunnel: ["Off" "High" "Medium" "Low"] -> w579
                frame "00", Default {
                }
                frame "01" {
                }
                frame "02" {
                }
                frame "04" {
                }
              }
              n147 = call "Build_ERD_Header_String_Array.vi"("ERD Name Array In"=w587, "ERD Number Array In"=w586, "ERD Name List"=string[] ["Signal Volume"], "New Header?"=w583, "ERD Number"=w581) -> ("ERD Name Array Out"=w585:string[], "ERD Number Array Out"=w584:string[])  [unwired: 13 in]
              n148 = Insert Into Array(array=w589, new element=w579) -> (w588:string[])  [unwired: 1 in]
              n149 = Bundle By Name(cluster=w593, "Signal Volume"=w579) -> (w592:T3)
            }
            frame 8272 {
              n150 = case shown="Default" w611 {
                selector: w611 -> [w614 _ _ _ _ _ _ _ _]
                tunnel: [w614 "Disabled" "No Heat" "Extra Low" "Low" "Medium" "High" "Max" "Don't Care"] -> w599
                frame Default {
                }
                frame "00" {
                }
                frame "01" {
                }
                frame "02" {
                }
                frame "03" {
                }
                frame "04" {
                }
                frame "05" {
                }
                frame "06" {
                }
                frame "07" {
                }
              }
              n151 = call "Build_ERD_Header_String_Array.vi"("ERD Name Array In"=w607, "ERD Number Array In"=w606, "ERD Name List"=string[] ["Temp Level"], "New Header?"=w601, "ERD Number"=w600) -> ("ERD Name Array Out"=w605:string[], "ERD Number Array Out"=w604:string[])  [unwired: 13 in]
              n152 = Insert Into Array(array=w603, new element=w599) -> (w602:string[])  [unwired: 1 in]
              n153 = Bundle By Name(cluster=w613, "Temp Level"=w599) -> (w612:T3)
            }
            frame 8269 {
              n154 = case shown="\"255\"" w637 {
                selector: w637 -> [w639 _ _ _ _ _ _ _ _]
                tunnel: [w639 "Disabled" "Damp" "Less Dry" "Dry" "More Dry" "Extra Dry" "Max" "Don't Care"] -> w624
                frame Default {
                }
                frame "00" {
                }
                frame "01" {
                }
                frame "02" {
                }
                frame "03" {
                }
                frame "04" {
                }
                frame "05" {
                }
                frame "06" {
                }
                frame "255" {
                }
              }
              n155 = call "Build_ERD_Header_String_Array.vi"("ERD Name Array In"=w632, "ERD Number Array In"=w631, "ERD Name List"=string[] ["Dryness Level"], "New Header?"=w628, "ERD Number"=w627) -> ("ERD Name Array Out"=w630:string[], "ERD Number Array Out"=w629:string[])  [unwired: 13 in]
              n156 = Insert Into Array(array=w626, new element=w624) -> (w625:string[])  [unwired: 1 in]
              n157 = Bundle By Name(cluster=w638, "Dryness Level"=w624) -> (w636:T3)
            }
            frame 8262 {
              n158 = call "HexStringToBoolean.vi"("Hex String"=w664) -> ("Boolean"=w649:bool)
              n159 = case shown="True" w649 {
                tunnel: ["OFF" "ON"] -> w659
                frame False {
                }
                frame True {
                }
              }
              n160 = Insert Into Array(array=w658, new element=w659) -> (w657:string[])  [unwired: 1 in]
              n161 = call "Build_ERD_Header_String_Array.vi"("ERD Name Array In"=w655, "ERD Number Array In"=w654, "ERD Name List"=string[] ["eDry"], "New Header?"=w651, "ERD Number"=w650) -> ("ERD Name Array Out"=w653:string[], "ERD Number Array Out"=w652:string[])  [unwired: 13 in]
              n162 = Bundle By Name(cluster=w663, "eDry"=w649) -> (w662:T3)
            }
            frame 61600 {
              n163 = call "HexStringToBoolean.vi"("Hex String"=w683) -> ("Boolean"=w668:bool)
              n164 = case shown="False" w668 {
                tunnel: ["OFF" "ON"] -> w678
                frame False {
                }
                frame True {
                }
              }
              n165 = Insert Into Array(array=w677, new element=w678) -> (w676:string[])  [unwired: 1 in]
              n166 = call "Build_ERD_Header_String_Array.vi"("ERD Name Array In"=w674, "ERD Number Array In"=w673, "ERD Name List"=string[] ["HeatControlRequest"], "New Header?"=w670, "ERD Number"=w669) -> ("ERD Name Array Out"=w672:string[], "ERD Number Array Out"=w671:string[])  [unwired: 13 in]
              n167 = Bundle By Name(cluster=w682, "HeatControl Request"=w668) -> (w681:T3)
            }
            frame 8311 {
              n168 = case shown="\"05\"" w700 {
                tunnel: ["TimeLevelOption_5" "TimeLevelOption_Disabled" "TimeLevelOption_1" "TimeLevelOption_2" "TimeLevelOption_3" "TimeLevelOption_4"] -> w687
                frame "05" {
                }
                frame "00", Default {
                }
                frame "01" {
                }
                frame "02" {
                }
                frame "03" {
                }
                frame "04" {
                }
              }
              n169 = call "Build_ERD_Header_String_Array.vi"("ERD Name Array In"=w695, "ERD Number Array In"=w694, "ERD Name List"=string[] ["Time Level"], "New Header?"=w691, "ERD Number"=w690) -> ("ERD Name Array Out"=w693:string[], "ERD Number Array Out"=w692:string[])  [unwired: 13 in]
              n170 = Insert Into Array(array=w689, new element=w687) -> (w688:string[])  [unwired: 1 in]
              n171 = Bundle By Name(cluster=w701, "Time Level"=w687) -> (w699:T3)
            }
            frame 8275 {
              n172 = call "HexStringToBoolean.vi"("Hex String"=w724) -> ("Boolean"=w709:bool)
              n173 = case shown="True" w709 {
                tunnel: ["OFF" "ON"] -> w719
                frame False {
                }
                frame True {
                }
              }
              n174 = Insert Into Array(array=w718, new element=w719) -> (w717:string[])  [unwired: 1 in]
              n175 = call "Build_ERD_Header_String_Array.vi"("ERD Name Array In"=w715, "ERD Number Array In"=w714, "ERD Name List"=string[] ["Extended Tumble"], "New Header?"=w711, "ERD Number"=w710) -> ("ERD Name Array Out"=w713:string[], "ERD Number Array Out"=w712:string[])  [unwired: 13 in]
              n176 = Bundle By Name(cluster=w723, "Ext. Tumble"=w709) -> (w722:T3)
            }
            frame 8266 {
              n177 = call "HexStringToBoolean.vi"("Hex String"=w743) -> ("Boolean"=w728:bool)
              n178 = case shown="True" w728 {
                tunnel: ["OFF" "ON"] -> w738
                frame False {
                }
                frame True {
                }
              }
              n179 = Insert Into Array(array=w737, new element=w738) -> (w736:string[])  [unwired: 1 in]
              n180 = call "Build_ERD_Header_String_Array.vi"("ERD Name Array In"=w734, "ERD Number Array In"=w733, "ERD Name List"=string[] ["Damp Alert"], "New Header?"=w730, "ERD Number"=w729) -> ("ERD Name Array Out"=w732:string[], "ERD Number Array Out"=w731:string[])  [unwired: 13 in]
              n181 = Bundle By Name(cluster=w742, "Damp Alert"=w728) -> (w741:T3)
            }
            frame 61501 {
              n182 = call "HexStringToBoolean.vi"("Hex String"=w762) -> ("Boolean"=w747:bool)
              n183 = case shown="True" w747 {
                tunnel: ["OFF" "ON"] -> w757
                frame False {
                }
                frame True {
                }
              }
              n184 = Insert Into Array(array=w756, new element=w757) -> (w755:string[])  [unwired: 1 in]
              n185 = call "Build_ERD_Header_String_Array.vi"("ERD Name Array In"=w753, "ERD Number Array In"=w752, "ERD Name List"=string[] ["Detangle"], "New Header?"=w749, "ERD Number"=w748) -> ("ERD Name Array Out"=w751:string[], "ERD Number Array Out"=w750:string[])  [unwired: 13 in]
              n186 = Bundle By Name(cluster=w761, "Detangle"=w747) -> (w760:T3)
            }
            frame 61503 {
              n187 = call "HexStringToBoolean.vi"("Hex String"=w779) -> ("Boolean"=w773:bool)
              n188 = case shown="True" w773 {
                tunnel: ["OFF" "ON"] -> w776
                frame False {
                }
                frame True {
                }
              }
              n189 = call "Build_ERD_Header_String_Array.vi"("ERD Name Array In"=w772, "ERD Number Array In"=w771, "ERD Name List"=string[] ["Delay Dry"], "New Header?"=w768, "ERD Number"=w766) -> ("ERD Name Array Out"=w770:string[], "ERD Number Array Out"=w769:string[])  [unwired: 13 in]
              n190 = Insert Into Array(array=w775, new element=w776) -> (w774:string[])  [unwired: 1 in]
              n191 = Bundle By Name(cluster=w781, "Delay Dry"=w773) -> (w780:T3)
            }
            frame 61510 {
              n192 = call "HexStringToBoolean.vi"("Hex String"=w798) -> ("Boolean"=w792:bool)
              n193 = case shown="True" w792 {
                tunnel: ["OFF" "ON"] -> w795
                frame False {
                }
                frame True {
                }
              }
              n194 = call "Build_ERD_Header_String_Array.vi"("ERD Name Array In"=w791, "ERD Number Array In"=w790, "ERD Name List"=string[] ["My Cycle"], "New Header?"=w787, "ERD Number"=w785) -> ("ERD Name Array Out"=w789:string[], "ERD Number Array Out"=w788:string[])  [unwired: 13 in]
              n195 = Insert Into Array(array=w794, new element=w795) -> (w793:string[])  [unwired: 1 in]
              n196 = Bundle By Name(cluster=w800, "My Cycle"=w792) -> (w799:T3)
            }
            frame 61609 {
              n197 = call "HexStringToBoolean.vi"("Hex String"=w819) -> ("Boolean"=w804:bool)
              n198 = call "Build_ERD_Header_String_Array.vi"("ERD Name Array In"=w813, "ERD Number Array In"=w812, "ERD Name List"=string[] ["TargetMoistureVoltageReached"], "New Header?"=w809, "ERD Number"=w808) -> ("ERD Name Array Out"=w811:string[], "ERD Number Array Out"=w810:string[])  [unwired: 13 in]
              n199 = case shown="True" w804 {
                tunnel: ["False" "True"] -> w805
                frame False {
                }
                frame True {
                }
              }
              n200 = Insert Into Array(array=w807, new element=w805) -> (w806:string[])  [unwired: 1 in]
              n201 = Bundle By Name(cluster=w818, "Target Voltage Reached"=w804) -> (w817:T3)
            }
            frame 61610 {
              n202 = case shown="\"00\", Default" w835 {
                tunnel: ["N/A" "Empty Drum" "Dry Load" "Cool Down Pasued" "Extended Tumble Paused" "Knob Change" "Power Button Pressed" "Cycle Completed"] -> w823
                frame "00", Default {
                }
                frame "01" {
                }
                frame "02" {
                }
                frame "03" {
                }
                frame "04" {
                }
                frame "05" {
                }
                frame "06" {
                }
                frame "07" {
                }
              }
              n203 = call "Build_ERD_Header_String_Array.vi"("ERD Name Array In"=w831, "ERD Number Array In"=w830, "ERD Name List"=string[] ["EOC Reason"], "New Header?"=w825, "ERD Number"=w824) -> ("ERD Name Array Out"=w829:string[], "ERD Number Array Out"=w828:string[])  [unwired: 13 in]
              n204 = Insert Into Array(array=w827, new element=w823) -> (w826:string[])  [unwired: 1 in]
              n205 = Bundle By Name(cluster=w837, "EOC Reason"=w823) -> (w836:T3)
            }
            frame 61823 {
              n206 = case shown="\"00\", Default" w859 {
                tunnel: ["IDLE" "NOT CONNECTED" "COMMISIONING" "COMMISIONING COMPLETE" "RECONNECTING" "CONNECTED"] -> w848
                frame "00", Default {
                }
                frame "01" {
                }
                frame "02" {
                }
                frame "03" {
                }
                frame "04" {
                }
                frame "05" {
                }
              }
              n207 = call "Build_ERD_Header_String_Array.vi"("ERD Name Array In"=w856, "ERD Number Array In"=w855, "ERD Name List"=w846, "New Header?"=w850, "ERD Number"=w849) -> ("ERD Name Array Out"=w854:string[], "ERD Number Array Out"=w853:string[])  [unwired: 13 in]
              n208 = Insert Into Array(array=w852, new element=w848) -> (w851:string[])  [unwired: 1 in]
              n209 = Bundle By Name(cluster=w861, "WiFiCommissioningPSt"=w848) -> (w860:T3)
            }
            frame 61615 {
              n210 = case shown="\"00\", Default" w881 {
                tunnel: ["Unknown" "Small" "Large"] -> w869
                frame "00", Default {
                }
                frame "01" {
                }
                frame "02" {
                }
              }
              n211 = call "Build_ERD_Header_String_Array.vi"("ERD Name Array In"=w877, "ERD Number Array In"=w876, "ERD Name List"=string[] ["LoadSizeByAggregation"], "New Header?"=w871, "ERD Number"=w870) -> ("ERD Name Array Out"=w875:string[], "ERD Number Array Out"=w874:string[])  [unwired: 13 in]
              n212 = Insert Into Array(array=w873, new element=w869) -> (w872:string[])  [unwired: 1 in]
              n213 = Bundle By Name(cluster=w883, "Load Size by Ag"=w869) -> (w882:T3)
            }
            frame 61613 {
              n214 = case shown="\"00\", Default" w900 {
                tunnel: ["Unknown" "Small" "Large"] -> w888
                frame "00", Default {
                }
                frame "01" {
                }
                frame "02" {
                }
              }
              n215 = call "Build_ERD_Header_String_Array.vi"("ERD Name Array In"=w896, "ERD Number Array In"=w895, "ERD Name List"=string[] ["Load by Temp"], "New Header?"=w890, "ERD Number"=w889) -> ("ERD Name Array Out"=w894:string[], "ERD Number Array Out"=w893:string[])  [unwired: 13 in]
              n216 = Insert Into Array(array=w892, new element=w888) -> (w891:string[])  [unwired: 1 in]
              n217 = Bundle By Name(cluster=w902, "Load Size by Temp"=w888) -> (w901:T3)
            }
            frame 61618 {
              n218 = case shown="\"00\", Default" w919 {
                tunnel: ["Undefined" "Small" "Large"] -> w907
                frame "00", Default {
                }
                frame "01" {
                }
                frame "02" {
                }
              }
              n219 = call "Build_ERD_Header_String_Array.vi"("ERD Name Array In"=w915, "ERD Number Array In"=w914, "ERD Name List"=string[] ["Vent Restriction"], "New Header?"=w909, "ERD Number"=w908) -> ("ERD Name Array Out"=w913:string[], "ERD Number Array Out"=w912:string[])  [unwired: 13 in]
              n220 = Insert Into Array(array=w911, new element=w907) -> (w910:string[])  [unwired: 1 in]
              n221 = Bundle By Name(cluster=w921, "Vent Restriction"=w907) -> (w920:T3)
            }
            frame 61617 {
              n222 = case shown="\"04\"" w938 {
                tunnel: ["Idle" "Disabled" "Phase 1Waiting" "Phase 2Waiting" "Phase 3Waiting" "Finished"] -> w926
                frame "00", Default {
                }
                frame "01" {
                }
                frame "02" {
                }
                frame "03" {
                }
                frame "04" {
                }
                frame "05" {
                }
              }
              n223 = call "Build_ERD_Header_String_Array.vi"("ERD Name Array In"=w934, "ERD Number Array In"=w933, "ERD Name List"=string[] ["Dry Load Detection"], "New Header?"=w928, "ERD Number"=w927) -> ("ERD Name Array Out"=w932:string[], "ERD Number Array Out"=w931:string[])  [unwired: 13 in]
              n224 = Insert Into Array(array=w930, new element=w926) -> (w929:string[])  [unwired: 1 in]
              n225 = Bundle By Name(cluster=w940, "Dry Load Detection"=w926) -> (w939:T3)
            }
            frame 61619 {
              n226 = case shown="\"01\"" w960 {
                tunnel: ["Disabled" "Idle" "Active" "Complete"] -> w948
                frame "00", Default {
                }
                frame "01" {
                }
                frame "02" {
                }
                frame "03" {
                }
              }
              n227 = call "Build_ERD_Header_String_Array.vi"("ERD Name Array In"=w956, "ERD Number Array In"=w955, "ERD Name List"=string[] ["Restriction Detection Status"], "New Header?"=w950, "ERD Number"=w949) -> ("ERD Name Array Out"=w954:string[], "ERD Number Array Out"=w953:string[])  [unwired: 13 in]
              n228 = Insert Into Array(array=w952, new element=w948) -> (w951:string[])  [unwired: 1 in]
              n229 = Bundle By Name(cluster=w962, "Restr Detect Status"=w948) -> (w961:T3)
            }
            frame 61624 {
              n230 = call "String Remove All Spaces.vi"("Input String"=w970) -> ("Spaces Removed"=w971:string)  [unwired: 13 in, 1 out]
              n231 = Hexadecimal String To Number(string=w971) -> (number=w968:u32)  [unwired: 2 in, 1 out]
              n232 = To Unsigned Word Integer(number=w968) -> (unsigned 16bit integer=w972:u16)
              n233 = Number To Decimal String(number=w968) -> (decimal integer string=w969:string)  [unwired: 1 in]
              n234 = call "Build_ERD_Header_String_Array.vi"("ERD Name Array In"=w980, "ERD Number Array In"=w979, "ERD Name List"=string[] ["Raw Moisture"], "New Header?"=w976, "ERD Number"=w975) -> ("ERD Name Array Out"=w978:string[], "ERD Number Array Out"=w977:string[])  [unwired: 13 in]
              n235 = Insert Into Array(array=w974, new element=w969) -> (w973:string[])  [unwired: 1 in]
              n236 = Bundle By Name(cluster=w985, "Raw Moisture"=w972) -> (w984:T3)
            }
            frame 61626 {
              n237 = case shown="\"08\"" w1000 {
                tunnel: ["Undefined" "Disabled" "Idle" "WaitForFilteredVoltageReset" "Sensing" "Paused" "PausedWhileWaitingForFilteredVoltageReset" "Target Reached" "TargetVoltageReachedByExpiredWatchdog"] -> w987
                frame "00", Default {
                }
                frame "01" {
                }
                frame "02" {
                }
                frame "03" {
                }
                frame "04" {
                }
                frame "05" {
                }
                frame "06" {
                }
                frame "07" {
                }
                frame "08" {
                }
              }
              n238 = call "Build_ERD_Header_String_Array.vi"("ERD Name Array In"=w995, "ERD Number Array In"=w994, "ERD Name List"=string[] ["Check Dampness State"], "New Header?"=w991, "ERD Number"=w990) -> ("ERD Name Array Out"=w993:string[], "ERD Number Array Out"=w992:string[])  [unwired: 13 in]
              n239 = Insert Into Array(array=w989, new element=w987) -> (w988:string[])  [unwired: 1 in]
              n240 = Bundle By Name(cluster=w1001, "Dampness State"=w987) -> (w999:T3)
            }
            frame 61731 {
              n241 = call "HexStringToBoolean.vi"("Hex String"=w1013) -> ("Boolean"=w1012:bool)
              n242 = case shown="True" w1012 {
                tunnel: ["OFF" "ON"] -> w1023
                frame False {
                }
                frame True {
                }
              }
              n243 = call "Build_ERD_Header_String_Array.vi"("ERD Name Array In"=w1019, "ERD Number Array In"=w1018, "ERD Name List"=string[] ["Steam Refresh"], "New Header?"=w1015, "ERD Number"=w1014) -> ("ERD Name Array Out"=w1017:string[], "ERD Number Array Out"=w1016:string[])  [unwired: 13 in]
              n244 = Insert Into Array(array=w1022, new element=w1023) -> (w1021:string[])  [unwired: 1 in]
              n245 = Bundle By Name(cluster=w1027, "Steam Refresh"=w1012) -> (w1026:T3)
            }
            frame 61743 {
              n246 = call "HexStringToBoolean.vi"("Hex String"=w1032) -> ("Boolean"=w1031:bool)
              n247 = case shown="True" w1031 {
                tunnel: ["OFF" "ON"] -> w1042
                frame False {
                }
                frame True {
                }
              }
              n248 = call "Build_ERD_Header_String_Array.vi"("ERD Name Array In"=w1038, "ERD Number Array In"=w1037, "ERD Name List"=string[] ["ReverseDrumInhibitRelay1"], "New Header?"=w1034, "ERD Number"=w1033) -> ("ERD Name Array Out"=w1036:string[], "ERD Number Array Out"=w1035:string[])  [unwired: 13 in]
              n249 = Insert Into Array(array=w1041, new element=w1042) -> (w1040:string[])  [unwired: 1 in]
              n250 = Bundle By Name(cluster=w1046, "ReverseDrumInhibitRelay1"=w1031) -> (w1045:T3)
            }
            frame 61744 {
              n251 = call "HexStringToBoolean.vi"("Hex String"=w1051) -> ("Boolean"=w1050:bool)
              n252 = case shown="True" w1050 {
                tunnel: ["OFF" "ON"] -> w1061
                frame False {
                }
                frame True {
                }
              }
              n253 = call "Build_ERD_Header_String_Array.vi"("ERD Name Array In"=w1057, "ERD Number Array In"=w1056, "ERD Name List"=string[] ["ReverseDrumInhibitRelay2"], "New Header?"=w1053, "ERD Number"=w1052) -> ("ERD Name Array Out"=w1055:string[], "ERD Number Array Out"=w1054:string[])  [unwired: 13 in]
              n254 = Insert Into Array(array=w1060, new element=w1061) -> (w1059:string[])  [unwired: 1 in]
              n255 = Bundle By Name(cluster=w1065, "ReverseDrumInhibitRelay2"=w1050) -> (w1064:T3)
            }
            frame 61956 {
              n256 = Decimal String To Number(string=w1085) -> (number=w1070:i32)  [unwired: 2 in, 1 out]
              n257 = To Unsigned Word Integer(number=w1070) -> (unsigned 16bit integer=w1069:u16)
              n258 = call "Build_ERD_Header_String_Array.vi"("ERD Name Array In"=w1079, "ERD Number Array In"=w1078, "ERD Name List"=string[] ["Raw Moisture"], "New Header?"=w1075, "ERD Number"=w1074) -> ("ERD Name Array Out"=w1077:string[], "ERD Number Array Out"=w1076:string[])  [unwired: 13 in]
              n259 = Number To Decimal String(number=w1070) -> (decimal integer string=w1073:string)  [unwired: 1 in]
              n260 = Insert Into Array(array=w1072, new element=w1073) -> (w1071:string[])  [unwired: 1 in]
              n261 = Bundle By Name(cluster=w1084, "Raw Moisture"=w1069) -> (w1083:T3)
            }
            frame 61719 {
              n262 = call "String Remove All Spaces.vi"("Input String"=w1088) -> ("Spaces Removed"=w1087:string)  [unwired: 13 in, 1 out]
              n263 = Hexadecimal String To Number(string=w1087) -> (number=w1090:u32)  [unwired: 2 in, 1 out]
              n264 = To Unsigned Word Integer(number=w1090) -> (unsigned 16bit integer=w1089:u16)
              n265 = call "Build_ERD_Header_String_Array.vi"("ERD Name Array In"=w1099, "ERD Number Array In"=w1098, "ERD Name List"=string[] ["MaxFilteredMoistureVoltageDuringASensingCycl"], "New Header?"=w1095, "ERD Number"=w1094) -> ("ERD Name Array Out"=w1097:string[], "ERD Number Array Out"=w1096:string[])  [unwired: 13 in]
              n266 = Number To Decimal String(number=w1090) -> (decimal integer string=w1093:string)  [unwired: 1 in]
              n267 = Insert Into Array(array=w1092, new element=w1093) -> (w1091:string[])  [unwired: 1 in]
              n268 = Bundle By Name(cluster=w1104, "MaxFIletered Voltage"=w1089) -> (w1103:T3)
            }
            frame 61968 {
              n269 = call "HexStringToBoolean.vi"("Hex String"=w1121) -> ("Boolean"=w1106:bool)
              n270 = call "Build_ERD_Header_String_Array.vi"("ERD Name Array In"=w1115, "ERD Number Array In"=w1114, "ERD Name List"=string[] ["Centrifugal Switch"], "New Header?"=w1111, "ERD Number"=w1110) -> ("ERD Name Array Out"=w1113:string[], "ERD Number Array Out"=w1112:string[])  [unwired: 13 in]
              n271 = case shown="True" w1106 {
                tunnel: ["OFF" "ON"] -> w1107
                frame False {
                }
                frame True {
                }
              }
              n272 = Insert Into Array(array=w1109, new element=w1107) -> (w1108:string[])  [unwired: 1 in]
              n273 = Bundle By Name(cluster=w1120, "Centrifugal Switch"=w1106) -> (w1119:T3)
            }
            frame 8193 {
              n274 = Hexadecimal String To Number(string=w1131) -> (number=w1132:u32)  [unwired: 2 in, 1 out]
              n275 = To Unsigned Word Integer(number=w1132) -> (unsigned 16bit integer=w1129:u16)
              n276 = case shown="0, Default" w1129 {
                tunnel: ["NotApplicable" "Drying" "MistSteam" "CoolDown" "ExtendedTumble" "Damp" "AirFluff"] -> w1126
                frame 0, Default {
                }
                frame 128 {
                }
                frame 129 {
                }
                frame 130 {
                }
                frame 131 {
                }
                frame 132 {
                }
                frame 133 {
                }
              }
              n277 = call "Build_ERD_Header_String_Array.vi"("ERD Name Array In"=w1138, "ERD Number Array In"=w1137, "ERD Name List"=w1124, "New Header?"=w1134, "ERD Number"=w1133) -> ("ERD Name Array Out"=w1136:string[], "ERD Number Array Out"=w1135:string[])  [unwired: 13 in]
              n278 = Insert Into Array(array=w1130, new element=w1126) -> (w1125:string[])  [unwired: 1 in]
              n279 = Bundle By Name(cluster=w1128, "Sub-Cycle"=w1126) -> (w1127:T3)
            }
            frame 63489..63508 {
              n280 = call "Build_ERD_Header_String_Array.vi"("ERD Name Array In"=w1161, "ERD Number Array In"=w1160, "ERD Name List"=string[] ["Min Sensing Eapse Time In Sec", "Time Multi Sec X 100", "Time Adder Sec"], "New Header?"=w1157, "ERD Number"=w1156) -> ("ERD Name Array Out"=w1159:string[], "ERD Number Array Out"=w1158:string[])  [unwired: 13 in]
              n281 = call "Parse Any Restric Data.vi"("Data"=w1153, "ERD_Always Show in"=w1155) -> ("CSV Data Out"=w1150:string[], "ERD_Always Show out"=w1154:T3)  [unwired: 7 in, 1 out]
              n282 = Insert Into Array(array=w1152, new element=w1150) -> (w1151:string[])  [unwired: 1 in]
            }
            frame 59 {
              n283 = call "VersionConversionData.vi"("Version In"=w1166) -> ("Version Out"=w1165:string)  [unwired: 9 in, 1 out]
              n284 = call "Build_ERD_Header_String_Array.vi"("ERD Name Array In"=w1173, "ERD Number Array In"=w1172, "ERD Name List"=string[] ["ParametricVersion"], "New Header?"=w1169, "ERD Number"=w1168) -> ("ERD Name Array Out"=w1171:string[], "ERD Number Array Out"=w1170:string[])  [unwired: 13 in]
              n285 = Bundle By Name(cluster=w1180, "Parametric Version"=w1165) -> (w1179:T2)
              n286 = Insert Into Array(array=w1176, new element=w1165) -> (w1175:string[])  [unwired: 1 in]
            }
            frame 61976 {
              n287 = case shown="\"02\"" w1184 {
                tunnel: ["APP" "Coin" "NotDefined"] -> w1181
                frame "01" {
                }
                frame "02" {
                }
                frame "00", Default {
                }
              }
              n288 = call "Build_ERD_Header_String_Array.vi"("ERD Name Array In"=w1189, "ERD Number Array In"=w1188, "ERD Name List"=w1187, "New Header?"=w1193, "ERD Number"=w1192) -> ("ERD Name Array Out"=w1191:string[], "ERD Number Array Out"=w1190:string[])  [unwired: 13 in]
              n289 = Bundle By Name(cluster=w1186, "Payment Method"=w1181) -> (w1185:T3)
              n290 = Insert Into Array(array=w1183, new element=w1181) -> (w1182:string[])  [unwired: 1 in]
            }
          }
          "Numeric" <- w40
        }
        n291 = in-place-cluster #1("CSV File String Arrays.ERD Name Array"=w21, "CSV File String Arrays.ERD Number Array"=w20, "Version"=w30, "ERD_Always Show"=w29, "Personality Set"=w27, "CSV File String Arrays.ERD Converted String Data"=w22, "Boot Loader Version"=w18) -> (w10:T1)
      }
    }
    frame Error {
      n292 = Unbundle By Name(w1202) -> ("code"=w1206:i32, "status"=w1207:bool, "source"=w1204:string)
      n293 = Equal?(x=w1206, y=-5006) -> (x = y?=w1210:bool)
      n294 = case shown="True" w1210 {
        tunnel: [w1214 FALSE] -> w1208
        tunnel: w1207 -> [w1214 _]
        tunnel: w1206 -> [w1213 w1216]
        tunnel: [w1213 w1216] -> w1205
        tunnel: [w1212 w1215] -> w1203
        tunnel: w1204 -> [w1212 w1215]
        frame False {
        }
        frame True {
        }
      }
      n295 = Bundle By Name(cluster=errorcluster {"status"=FALSE, "code"=0, "source"=""} ("error constant"), "status"=w1208, "code"=w1205, "source"=w1203) -> (w1201:errorcluster)
    }
  }
  "Error Out" <- w5
  "All_ERD_Data_Bundled_Brass" <- w1
